vi "Init Device.vi"() -> ()   [LabVIEW 2011, in "LVH-LINX.lvlib"]
uses:
  <vilib>/LabVIEW Hacker/LINX/LVH-LINX.lvlib
  <vilib>/LabVIEW Hacker/LINX/Private/Type Defs/User Platform.ctl
panel:
  in  "Platform":T1
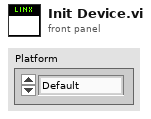
[diagram p1: front panel]
types:
  T1 = typedef "LVH-LINX.lvlib/User Platform.ctl" = enum16{"Default", "LINX", "myRIO"}
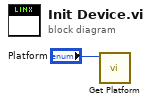
[diagram p0: block diagram]
diagram:
  n1 = call <vilib>:"Get Platform.vi"("Platform"="Platform") -> ()  [unwired: 10 in, 1 out]
